vi "Summarise FFT.vi"(9 "dB cutoff":dbl[](array[numeric])=[-3.0, -6.0, -9.0], 10 "df":dbl=0.07322788517867605, 11 "Power Spectrum (V^2 rms)":dbl[](array[numeric])=array[5121 elements]) -> (1 "peaks found":i32, 2 "Dominant freqs":T1(array[cluster]), 3 "Cuttoff freqs":cluster{"dB cutoff":dbl, "freqs":dbl[]}[](array[cluster])=[{"dB cutoff"=-3.0, "freqs"=[nan, nan]}, {"dB cutoff"=-6.0, "freqs"=[nan, nan]}, {"dB cutoff"=-9.0, "freqs"=[nan, nan]}])   [LabVIEW 2016]
uses:
  <vilib>/Analysis/NI_AAL_SigProc.lvlib
panel:
  out "Power Spectrum (dB)":cluster{"Time":dbl[], "Data":dbl[]}(graph)
  out "Power (RMS)":cluster{"Time":dbl[], "Data":dbl[]}(graph)
  in  "width":i32=3 min=3
  in  "threshold":dbl(slide) scale=-10.0..10.0
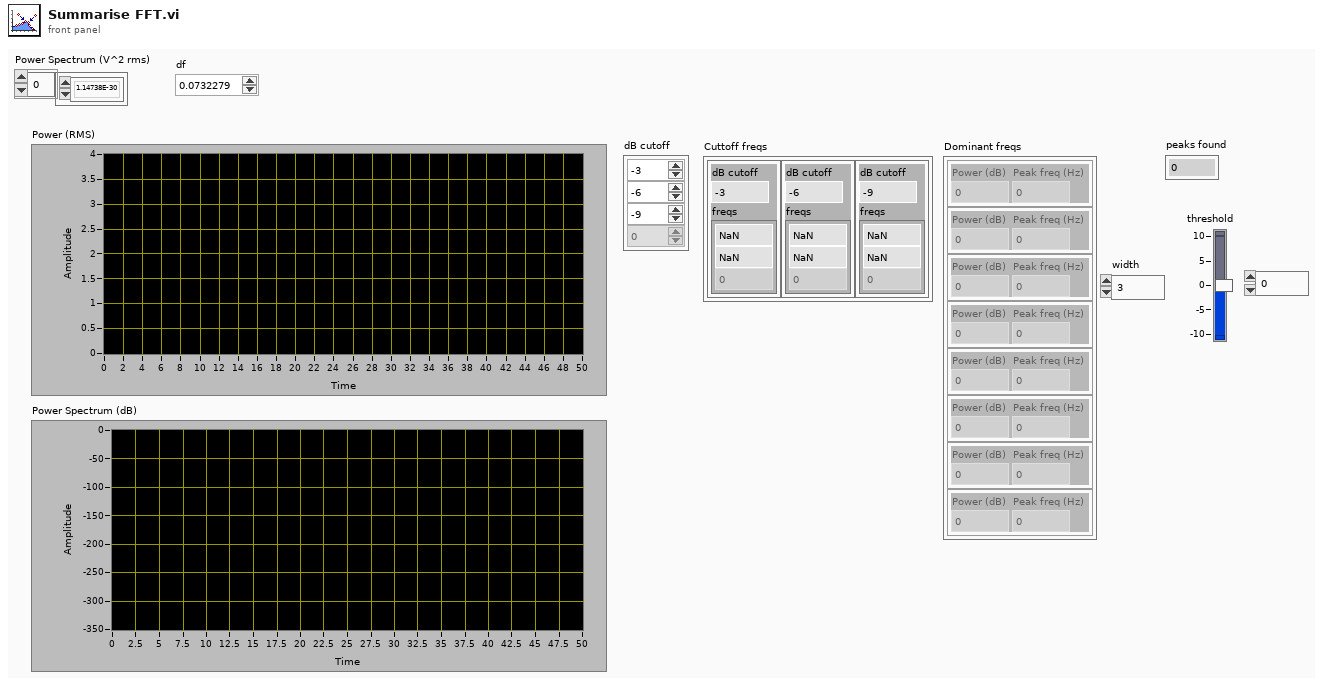
[diagram p1: front panel]
types:
  T1 = cluster{"Power (dB)":dbl, "Peak freq (Hz)":dbl}[]
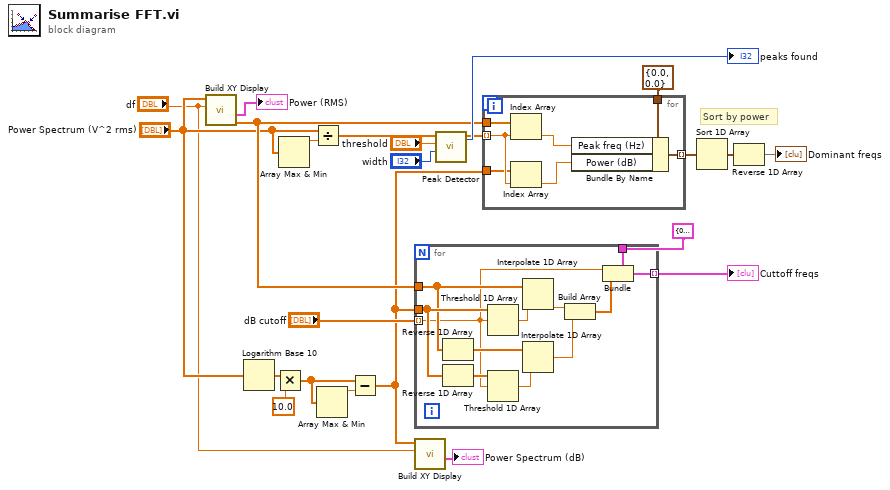
[diagram p0: block diagram]
diagram:
  # "Sort by power"
  n1 = call <userlib>:"Build XY Display.vi"("dt"="df", "Data"="Power Spectrum (V^2 rms)") -> ("Time"=w10:dbl[], "Data"=→"Power (RMS)":cluster{"Time":dbl[], "Data":dbl[]})  [unwired: 6 in, 2 out]
  n2 = Logarithm Base 10(1:"Power Spectrum (V^2 rms)") -> (0:w13:dbl[])
  n3 = Multiply(x=w13, y=10.0) -> (x*y=w12:dbl[])
  n4 = Array Max & Min(array="Power Spectrum (V^2 rms)") -> (max value=w18:dbl)  [unwired: 3 out]
  n5 = Divide(x="Power Spectrum (V^2 rms)", y=w18) -> (x/y=w17:dbl[])
  n6 = Array Max & Min(array=w12) -> (max value=w11:dbl)  [unwired: 3 out]
  n7 = Subtract(x=w12, y=w11) -> (x-y=w6:dbl[])
  n8 = for {
    tunnel: "dB cutoff" -> [w26] mode=indexing
    tunnel: w6 -> [w33]
    tunnel: w10 -> [w32]
    tunnel: [w25] -> w22 mode=indexing
    tunnel: cluster{"dB cutoff":dbl, "freqs":dbl[]} {"dB cutoff"=0.0, "freqs"=[]} -> [w24]
    n9 = Reverse 1D Array(array=w32) -> (reversed array=w31:dbl[])
    n10 = Reverse 1D Array(array=w33) -> (reversed array=w34:dbl[])
    n11 = Threshold 1D Array(2:w26, 3:w33) -> (0:w35:dbl)  [unwired: 1 in]
    n12 = Threshold 1D Array(2:w26, 3:w34) -> (0:w30:dbl)  [unwired: 1 in]
    n13 = Interpolate 1D Array(1:w35, 2:w32) -> (0:w29:dbl)
    n14 = Interpolate 1D Array(1:w30, 2:w31) -> (0:w28:dbl)
    n15 = Build Array(w29, w28) -> (w27:dbl[])
    n16 = Bundle(cluster=w24, "dB cutoff"=w26, "freqs"=w27) -> (w25:cluster{"dB cutoff":dbl, "freqs":dbl[]})
  }
  "Cuttoff freqs" <- w22
  n17 = call <userlib>:"Build XY Display.vi"("dt"="df", "Data"=w6) -> ("Data"=→"Power Spectrum (dB)":cluster{"Time":dbl[], "Data":dbl[]})  [unwired: 6 in, 3 out]
  n18 = call <vilib>:"Peak Detector.vi"("width"="width", "threshold"="threshold", "X"=w17) -> ("Locations"=w16:dbl[], "# found"=→"peaks found":i32)  [unwired: 4 in, 3 out]
  n19 = for {
    tunnel: w10 -> [w42]
    tunnel: w16 -> [w41] mode=indexing
    tunnel: w6 -> [w40]
    tunnel: [w39] -> w7 mode=indexing
    tunnel: cluster{"Power (dB)":dbl, "Peak freq (Hz)":dbl} {"Power (dB)"=0.0, "Peak freq (Hz)"=0.0} -> [w38]
    n20 = Index Array(array=w42, index=w41) -> (element=w36:dbl)
    n21 = Index Array(array=w40, index=w41) -> (element=w37:dbl)
    n22 = Bundle By Name(cluster=w38, "Peak freq (Hz)"=w36, "Power (dB)"=w37) -> (w39:cluster{"Power (dB)":dbl, "Peak freq (Hz)":dbl})
  }
  n23 = Sort 1D Array(array=w7) -> (sorted array=w3:T1)
  n24 = Reverse 1D Array(array=w3) -> (reversed array=→"Dominant freqs":T1)
